vi "AVTCP-Filepath FGV.vi"(4 "Value in":path, 5 "Action":T1=enum."Read") -> (0 "Value out":path)   [LabVIEW 2020]
uses:
  AVTCP-FGV Action.ctl
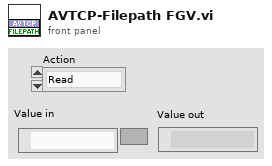
[diagram p1: front panel]
types:
  T1 = typedef "AVTCP-FGV Action.ctl" = enum16{"Init", "Write", "Read"}
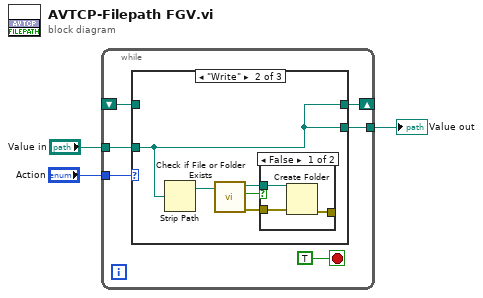
[diagram p0: block diagram]
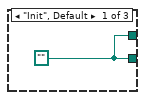
[diagram p2: hidden frame]
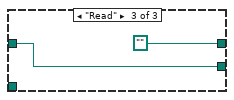
[diagram p4: hidden frame]
diagram:
  n1 = while {
    tunnel: "Action" -> [w9]
    tunnel: "Value in" -> [w7]
    shift-right: [w8] -> _
    shift-left: _ -> [w6]
    tunnel: [w5] -> w1
    stop <- TRUE stop-if-true
    n2 = case shown="\"Write\"" w9 {
      tunnel: [w10 w15 path ""] -> w8
      tunnel: w7 -> [_ w15 _]
      tunnel: w6 -> [_ _ w20]
      tunnel: [w10 w15 w20] -> w5
      frame "Init", Default {
        w10 = path ""
      }
      frame "Write" {
        n3 = Strip Path(path=w15) -> (stripped path=w14:path)  [unwired: 1 out]
        n4 = call <vilib>:"Check if File or Folder Exists.vi"("path"=w14) -> ("error out"=w11:errorcluster, "file or folder exists?"=w13:bool, "dup path"=w12:path)  [unwired: 8 in]
        n5 = case shown="False" w13 {
          tunnel: w12 -> [w18 _]
          tunnel: w11 -> [w17 _]
          tunnel: [w16 _] -> _
          frame False {
            n6 = Create Folder(path (use dialog)=w18, error in=w17) -> (error out=w16:errorcluster)  [unwired: 1 in, 2 out]
          }
          frame True {
          }
        }
      }
      frame "Read" {
      }
    }
  }
  "Value out" <- w1
